vi "Set Alarm Color.vi"(10 "Warning":bool[](array[boolean]), 11 "Fault":bool[](array[boolean])) -> (3 "Alarm color":T1=[{16711680, 0}, {0, 0}])   [LabVIEW 2015, in "Utility.lvlib"]
uses:
  Utility.lvlib
  Alarm Color.ctl
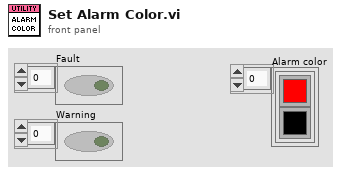
[diagram p1: front panel]
types:
  T1 = typedef "Utility.lvlib/Alarm Color.ctl" = cluster{u32, u32}[]
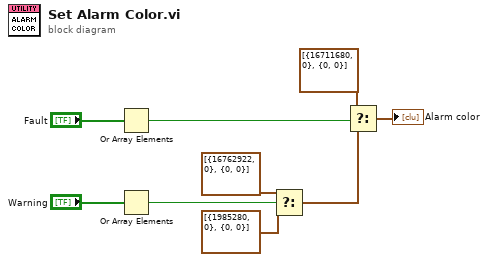
[diagram p0: block diagram]
diagram:
  n1 = Or Array Elements(Boolean array="Fault") -> (logical OR=w4:bool)
  n2 = Or Array Elements(Boolean array="Warning") -> (logical OR=w1:bool)
  n3 = Select(t=T1 [{16762922, 0}, {0, 0}] ("Colors [4]"), s=w1, f=T1 [{1985280, 0}, {0, 0}] ("Colors [4]")) -> (s? t:f=w8:T1)
  n4 = Select(t=T1 [{16711680, 0}, {0, 0}] ("Colors [4]"), s=w4, f=w8) -> (s? t:f=→"Alarm color":T1)
